vi "test-30frame-QR-static.vi"() -> ()   [LabVIEW 2015]
uses:
  <vilib>/Utility/error.llb/whitespace.ctl
  <vilib>/MakerHub/LINX/Public/Peripherals/Digital/Digital Write 1 Chan.vi
  <vilib>/MakerHub/LINX/Public/Peripherals/Analog/Analog Read N Chans.vi
  <vilib>/MakerHub/LINX/Public/Peripherals/Digital/Digital Write N Chans.vi
  <vilib>/MakerHub/LINX/Private/Local IO/LinxAnalogRead.vi
  <vilib>/MakerHub/LINX/Public/Utilities/Check Channel.vi
  <vilib>/MakerHub/LINX/Private/Local IO/LinxDigitalWrite.vi
  <vilib>/Instr/_visa.llb/VISA Configure Serial Port (Instr).vi
  <vilib>/MakerHub/LINX/Public/Utilities/Open Serial.vi
  <vilib>/MakerHub/LINX/Private/Utilties/Generate Error.vi
  <vilib>/ptbypt/NI_PtbyPt.lvlib
  <vilib>/MakerHub/LINX/LMH-LINX.lvlib
panel:
  out "gat hang 2":bool
  in  "measurement":dbl
  in  "calculate":dbl
  out "Appear":bool
  out "gat hang":bool
  in  "?":T1(tab)=enum."CONTROL & SUPERVISORY"
  in  "?":i32(listbox)
  out "Form QR ?":bool
  out "Data#":bool
  out "Found?":bool
  out "False Package":dbl
  out "SS3":bool=TRUE
  out "SS2":bool=TRUE
  out "SS1":bool=TRUE
  out "Processing Chart":cluster{dbl, dbl, dbl, dbl, "mean":dbl}(graph)={0.0, 0.0, 0.0, -16.408877733961745, "mean"=-16.408877733961745}
  out "WEIGHT PASS":bool
  out "Calculate\nValue":dbl
  out "DATA":string
  out "QR PASS":bool
  out "Well Package":i32
  out "Measurement\nValue":dbl format="%#.3f"
  in  "zero":bool
  in  "No. Accurate (g)":dbl=10.0 format="%#_13g"
  in  "Fillter":bool
  in  "STOP":bool
  in  "Start measurement":bool caption="Ðo tuyÌ choòn"
  out "CTHT1":bool=TRUE
  out "CTHT2":bool=TRUE
  in  "button CTHT 2":bool
  in  "button CTHT 1":bool
  in  "button SS 3":bool
  in  "button SS 2":bool
  in  "button SS 1":bool
  out "Trigger1":bool
  out "Trigger 2":bool
  out "?":T2(plugin-control)
  out "S/N":string
  out "C/N":string
  out "Run Loop":i32=777
  in  "Sensor Channels":u8[](array[numeric])=[4, 5, 6, 0, 1]
  in  "Path save data report":path=path "C:/Data"
  in  "COM Port Controller":refnum<visa-resource-name>="COM18"
  out "Quantity":i32=35
  out "Mass (kg):":dbl=2.0
  out "Tong K/lg (kg)":dbl=70.0
  in  "VISA resource name":refnum<visa-resource-name>="COM12"
  out "Array":i32[](array[numeric])
  out "Numeric 2":i32=233
  out "Raw data":dbl
  out "Fine Data":dbl=-16.408877733961745
  in  "zero":dbl=16.408877733961745
  in  "he so calib":dbl=8.552828494462736 format="%#_12g"
  in  "Serial Settings":T3={"baud rate"=19200, "data bits"=8, "parity"=enum."None", "stop bits"=10, "flow control"=0} {"flow control" items=["None"=0, "XON/XOFF"=1, "RTS/CTS"=2, "DTR/DSR"=4]; "stop bits" items=["1.0"=10, "1.5"=15, "2.0"=20]; "data bits" min=5 max=8 step=1; "baud rate" items=["75"=75, "110"=110, "134"=134, "150"=150, "300"=300, "600"=600, "1200"=1200, "1800"=1800, "2400"=2400, "4800"=4800, "7200"=7200, "9600"=9600, "14400"=14400, "19200"=19200, "28800"=28800, "38400"=38400, "56000"=56000, "57600"=57600, "115200"=115200, "128000"=128000, "230400"=230400]}
  in  "Low factor":cluster{"1":dbl, "2":dbl, "3":dbl}={"1"=177000.0, "2"=222000.0, "3"=-207250.0}
  in  "High Factor":cluster{"1":dbl, "2":dbl, "3":dbl}={"1"=1073000.0, "2"=1137000.0, "3"=703000.0} {"3" format="%#_15f"}
  in  "Termination Character":u8=10 format="%.0x"
  in  "End Read on\n Termination Character?":bool=TRUE
  in  "index":i32
  in  "sample length":i32=100
  in  "Numeric":i32=500
  in  "Pulse pin 2":u8=7
  in  "DIR pin 2":u8=6
  out "notifier out":refnum<notifier>
  in  "V-ref-trigger":dbl=0.2 format="%#_13g"
  out "Sensors Chart":T4(graph)={"Voltages[0]"=2.9833984375, "Voltages[1]"=1.728515625, "Voltages[2]"=0.9033203125, "Voltages[3]"=4.228515625, "Voltages[4]"=4.27734375, "Voltages[5]"=0.0, "Voltages[6]"=0.0, "Voltages[7]"=0.0, "Voltages[8]"=0.0}
  in  "Enable pin 2":u8=5
  in  "Frequency (Hz) 2":u32=6400
  in  "Frequency (Hz)":u32=6400
  in  "Pulse pin":u8=4
  in  "DIR pin":u8=3
  in  "enable pin":u8=2
  # "HÊò THÔìNG KIÊÒM TRA CHÂìT LÝÕòNG ÐOìNG GOìI THUÌNG HAÌNG\n THEO MAÞ QR & ÌKHÔìI LÝÕòNG"
  # "Table Result"
  # "TEST"
  # "Sensors"
  # "Control"
  # "Weight Transmit"
  # "Motor1"
  # "Motor2"
  # "Image Processing"
  # "Report"
  # "Distance Sensors and Limit Switch"
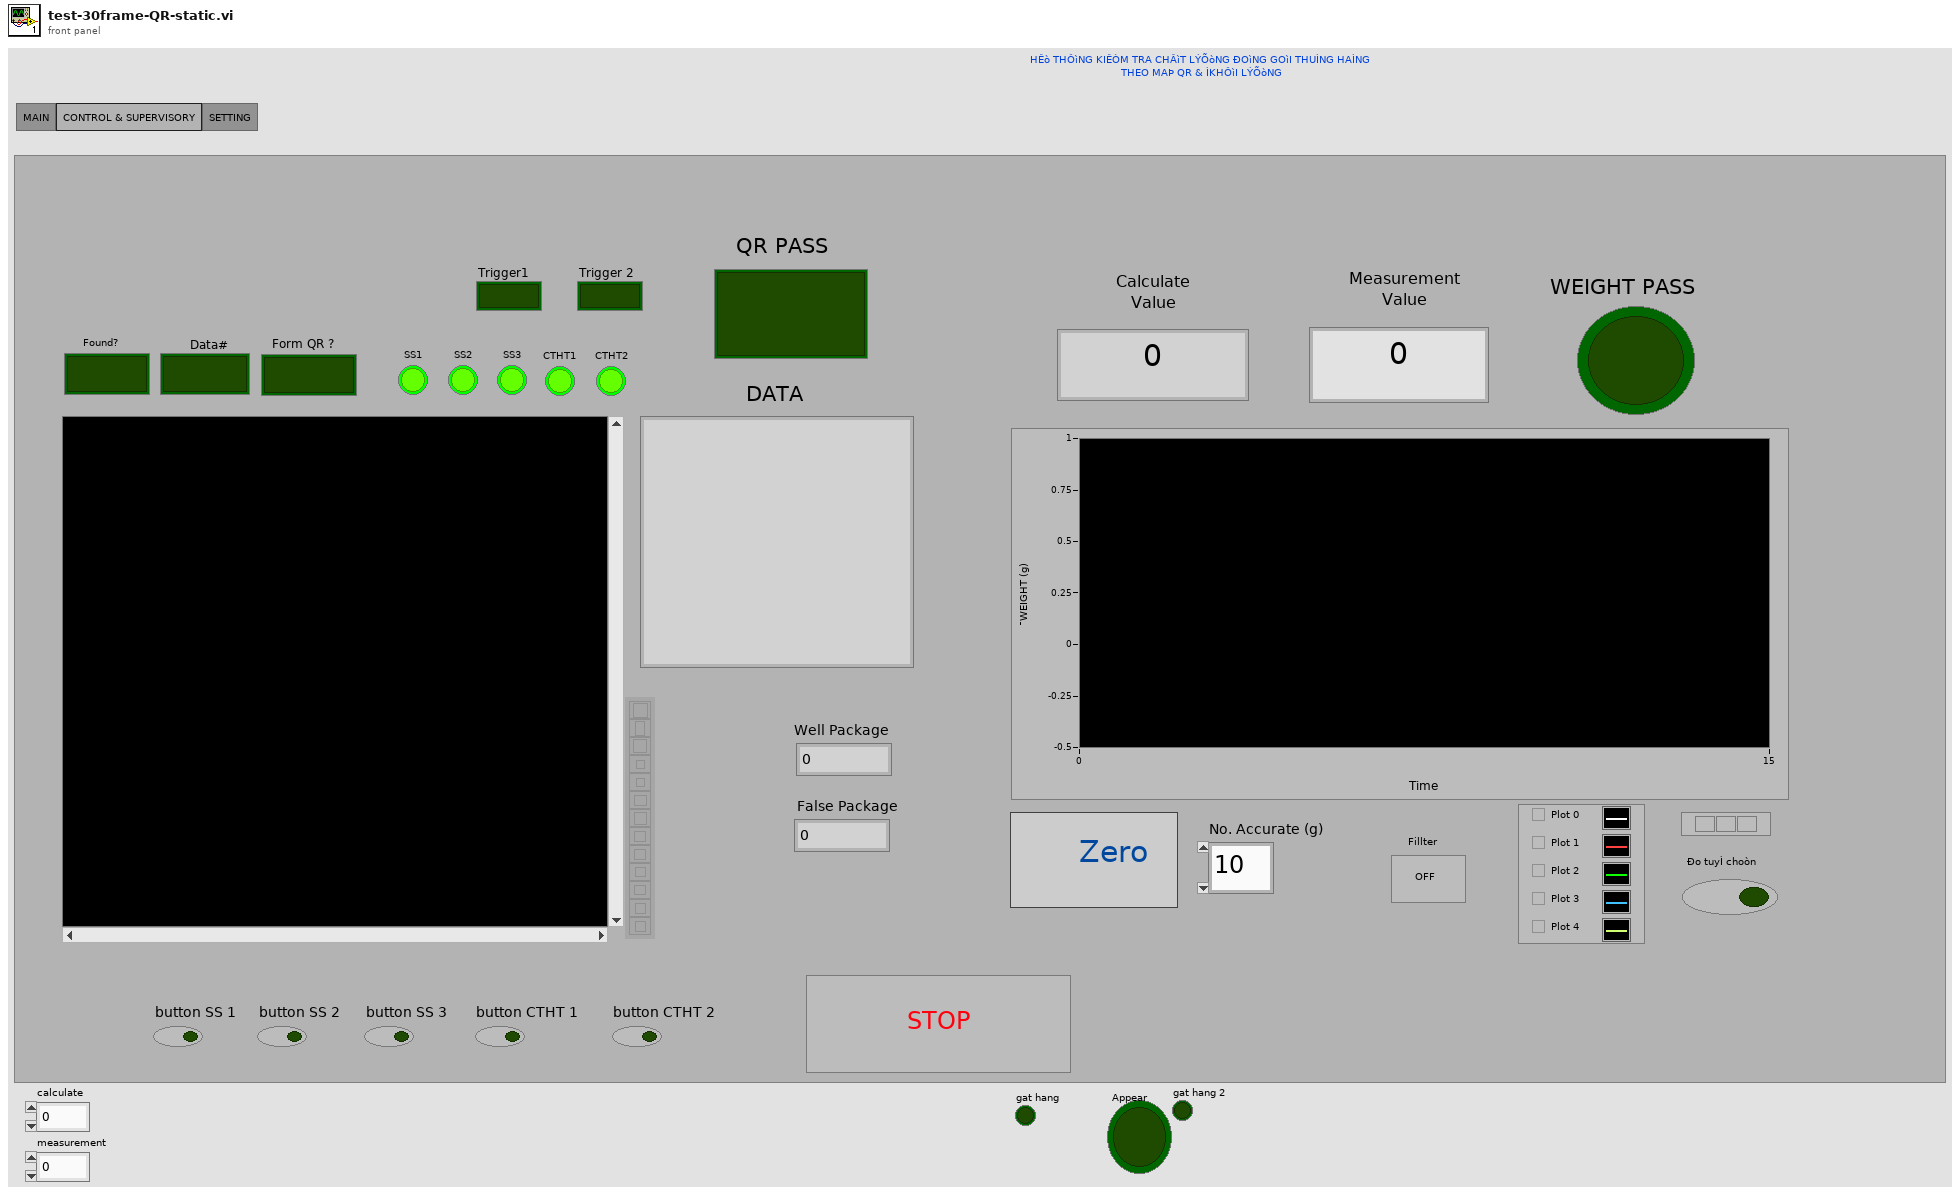
[diagram p1: front panel]
types:
  T1 = enum32{"MAIN", "CONTROL & SUPERVISORY", "SETTING"}
  T2 = typedef "IMAQ Image.ctl" = refnum<image>
  T3 = cluster{"baud rate":u32, "data bits":u16, "parity":enum16{"None", "Odd", "Even", "Mark", "Space"}, "stop bits":u16, "flow control":u16}
  T4 = cluster{"Voltages[0]":dbl, "Voltages[1]":dbl, "Voltages[2]":dbl, "Voltages[3]":dbl, "Voltages[4]":dbl, "Voltages[5]":dbl, "Voltages[6]":dbl, "Voltages[7]":dbl, "Voltages[8]":dbl}
  T5 = typedef "LMH-LINX.lvlib/LINX Ref.ctl" = cluster{"IO":T6, "Interface":T7, "LINX Device Config":T8}
  T6 = typedef "LMH-LINX.lvlib/Platform.ctl" = enum16{"Remote", "Local"}
  T7 = typedef "LMH-LINX.lvlib/Interface.ctl" = enum16{"Serial", "TCP"}
  T8 = typedef "LMH-LINX.lvlib/Device.lvlib/LINX Device Config.ctl" = cluster{"Interface":T7, "COM Port":refnum<visa-resource-name>, "TCP Configuration":T9, "Device Family":u8, "Device ID":u8, "Device Name":string, "TCP Ref":refnum<k5>, "Channels":T10}
  T9 = typedef "LMH-LINX.lvlib/Device.lvlib/TCP Config.ctl" = cluster{"IP Address":string, "Port":u16}
  T10 = typedef "LMH-LINX.lvlib/Channels.ctl" = cluster{"DI":u8[], "DO":u8[], "AI":u8[], "AO":u8[], "PWM":u8[], "QE":u8[], "UART":u8[], "I2C 2":u8[], "SPI":u8[], "CAN":u8[], "Servo":u8[], "AI Ref (V)":dbl, "AI Resolution (Bits)":u8, "AO Ref (V)":dbl, "AO Resolution (Bits)":u8}
  T11 = typedef "whitespace.ctl" = u16
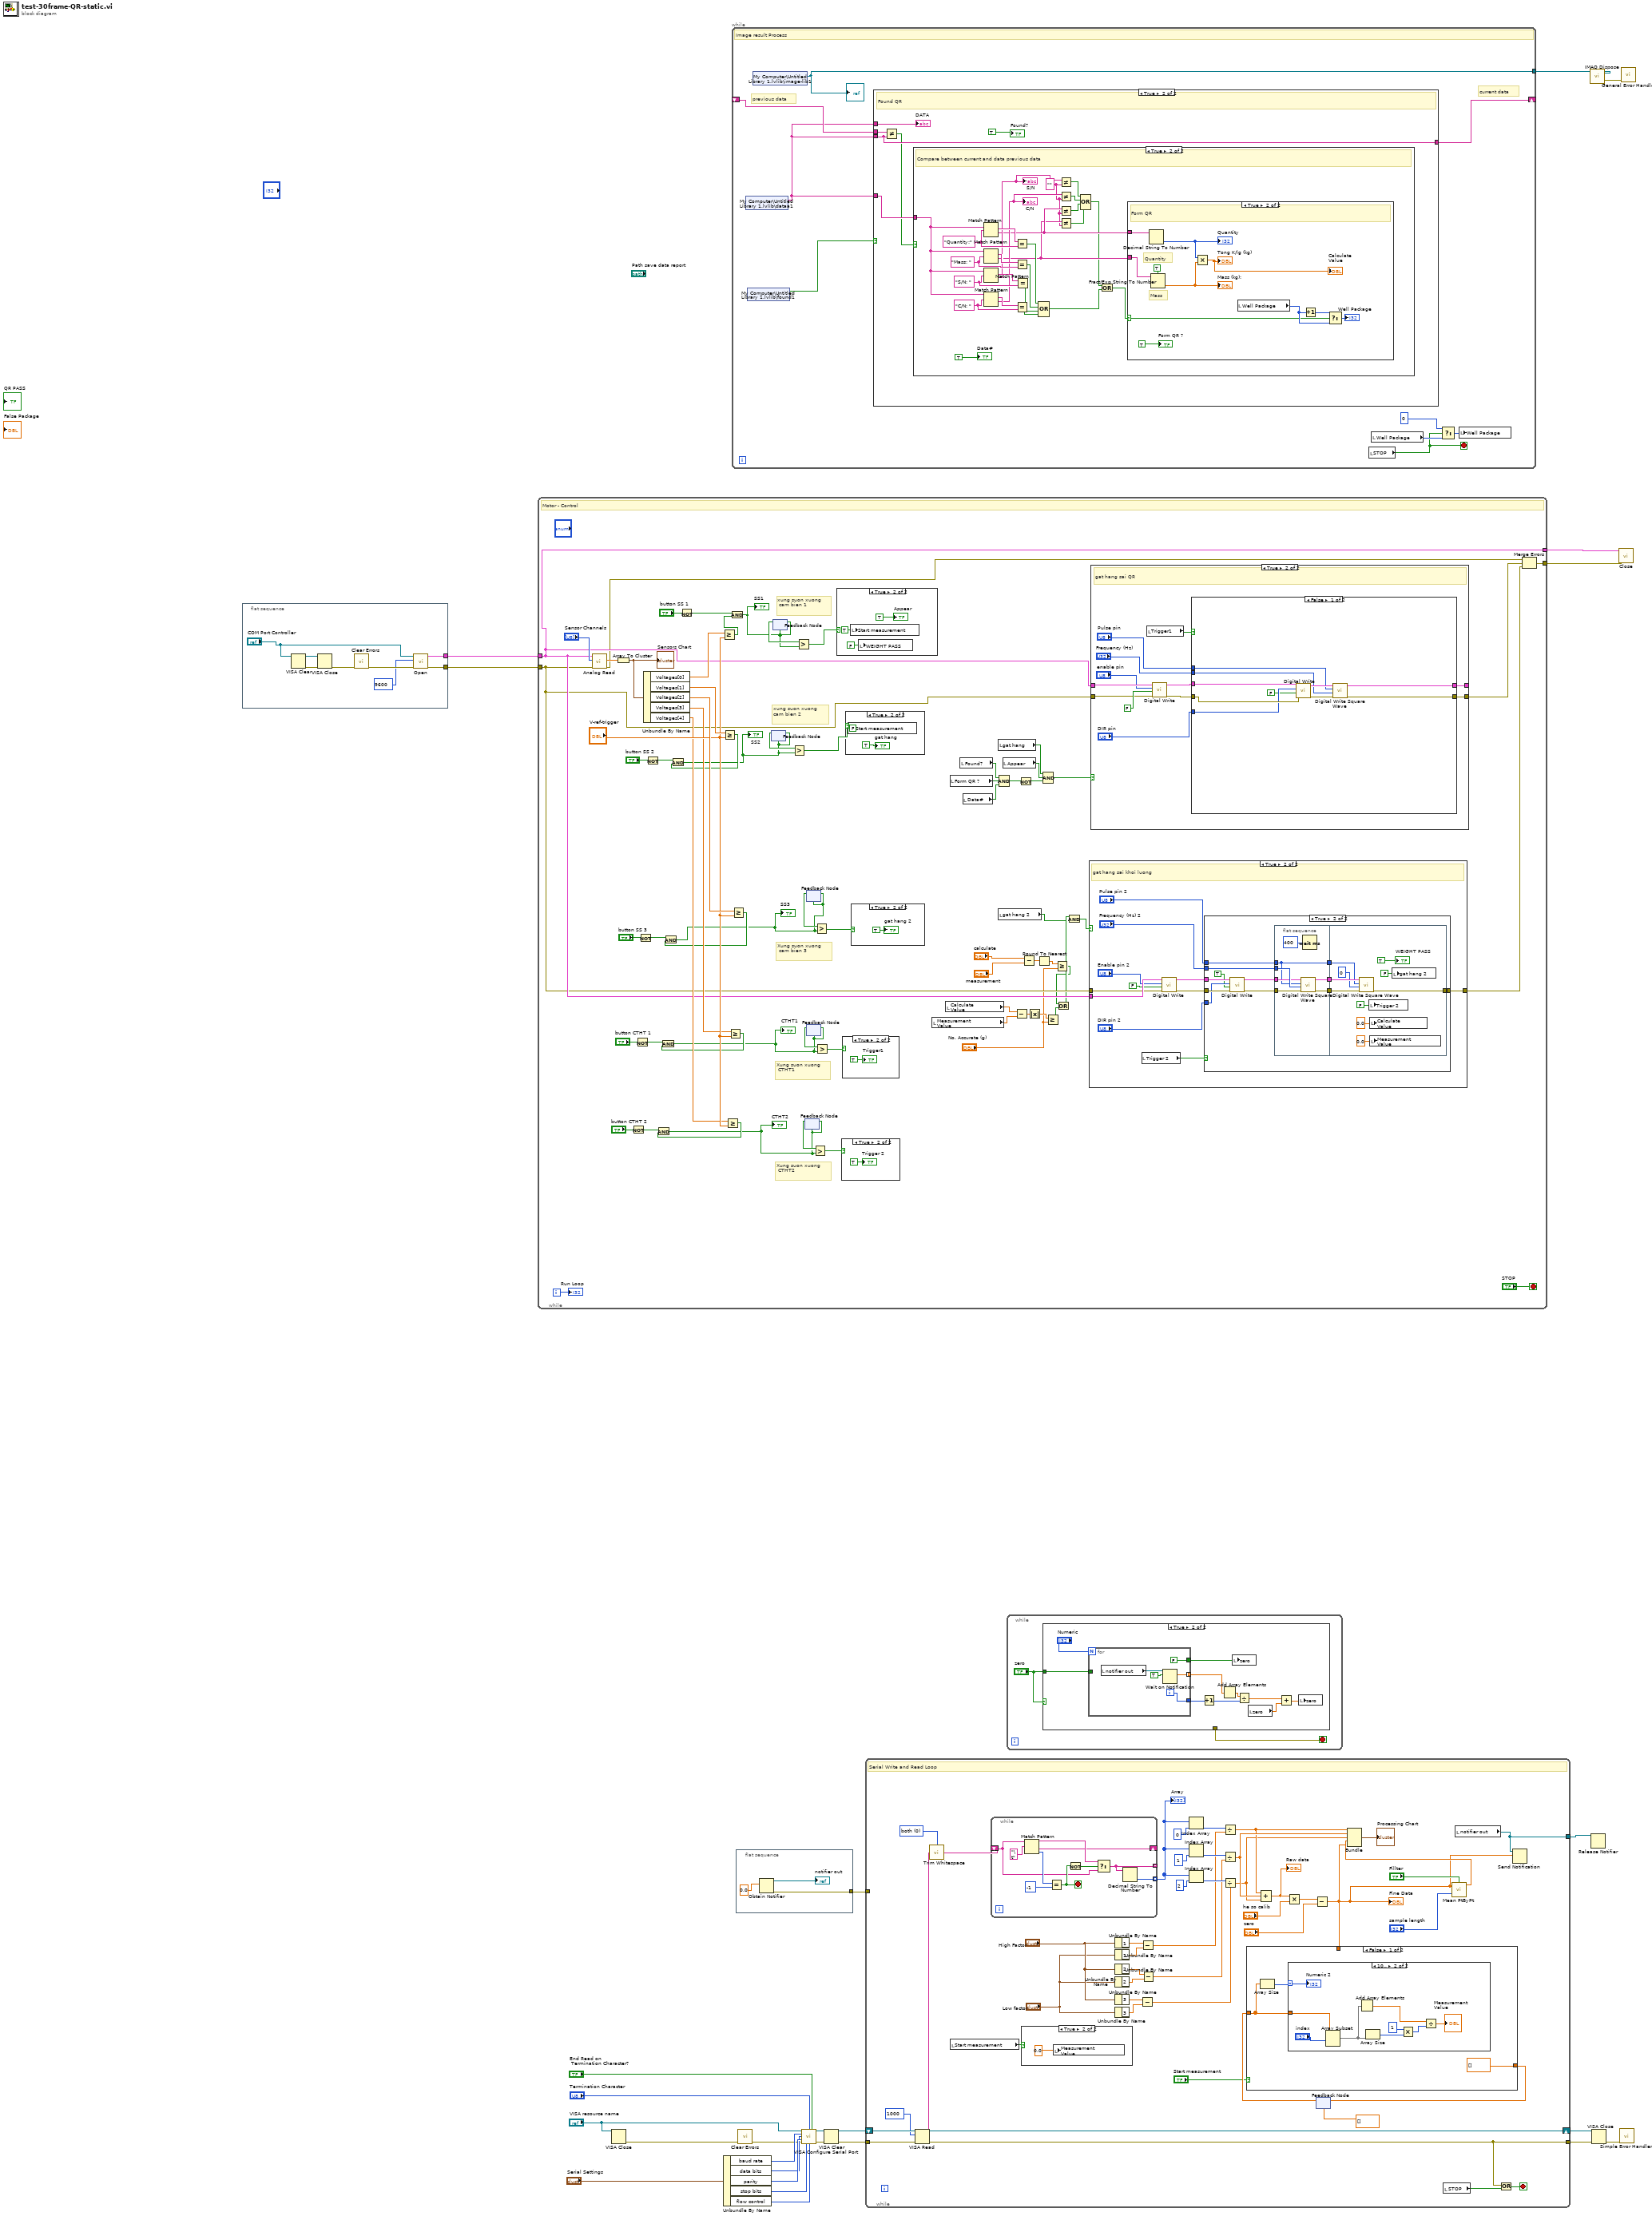
[diagram p0: block diagram]
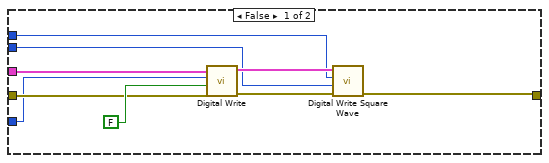
[diagram p7: hidden frame]
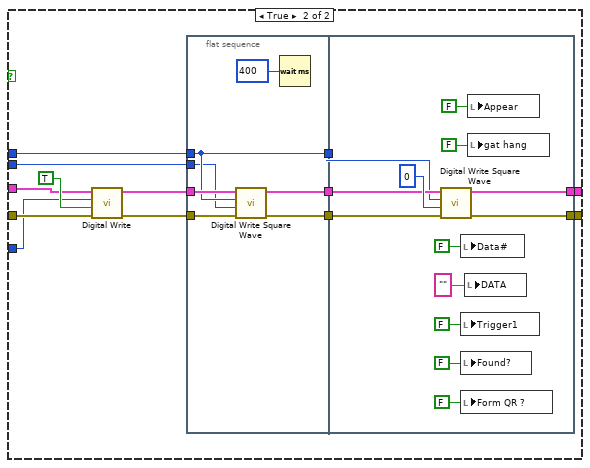
[diagram p11: hidden frame]
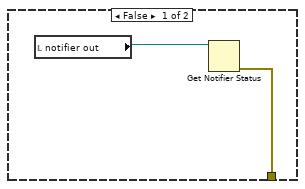
[diagram p14: hidden frame]
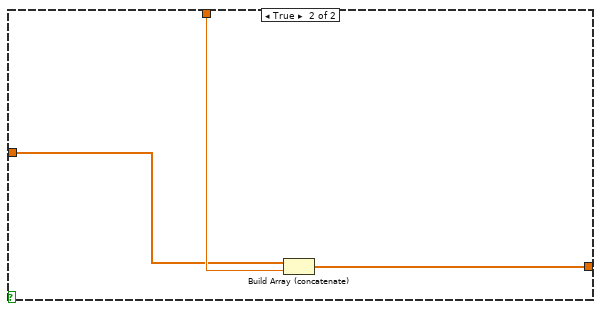
[diagram p17: hidden frame]
diagram:
  n1 = flat-sequence {
    tunnel: [w32] -> w2
    tunnel: [w31] -> w1
    frame #0 {
      n2 = VISA Clear(VISA resource name="COM Port Controller") -> (VISA resource name out=w29:refnum<visa-resource-name>, error out=w27:errorcluster)  [unwired: 1 in]
      n3 = VISA Close(VISA resource name=w29, error in (no error)=w27) -> (error out=w34:errorcluster)
      n4 = call <vilib>:"Clear Errors.vi"("error in (no error)"=w34) -> ("error out"=w33:errorcluster)  [unwired: 5 in, 1 out]
      n5 = call-poly <vilib>:"Open.vi"("Error In"=w33, "Baud Rate Override"=u32 9600, "Serial Port"="COM Port Controller") -> ("Error Out"=w31:errorcluster, "LINX Resource"=w32:T5)  [unwired: 6 in, 1 out]
    }
  }
  n6 = while {
    tunnel: w2 -> [w61]
    tunnel: w1 -> [w60]
    tunnel: [w56] -> w4
    tunnel: [w61] -> w3
    i -> [w101]
    stop <- "STOP" stop-if-true
    # "Xung suon xuong\n CTHT2"
    # "Xung suon xuong\n CTHT1"
    # "xung suon xuong\n cam bien 1"
    # "Xung suon xuong\n cam bien 3"
    # "xung suon xuong \ncam bien 2"
    # "Motor - Control"
    n7 = call-poly <vilib>:"Analog Read.vi"("Error In"=w60, "AI Channel(s)"="Sensor Channels", "LINX Resource"=w61) -> ("Error Out"=w55:errorcluster, "Voltages"=w103:dbl[])  [unwired: 5 in, 2 out]
    n8 = Array To Cluster(array=w103) -> (cluster=w92:T4)
    "Sensors Chart" <- w92
    n9 = Not(x="button CTHT 2") -> (.not. x?=w74:bool)
    n10 = Not(x="button CTHT 1") -> (.not. x?=w76:bool)
    n11 = Not(x="button SS 3") -> (.not. x?=w80:bool)
    n12 = Unbundle By Name(w92) -> ("Voltages[0]"=w99:dbl, "Voltages[1]"=w98:dbl, "Voltages[2]"=w97:dbl, "Voltages[3]"=w88:dbl, "Voltages[4]"=w87:dbl)
    n13 = Not(x="button SS 2") -> (.not. x?=w82:bool)
    n14 = Not(x="button SS 1") -> (.not. x?=w84:bool)
    n15 = Greater Or Equal?(x=w99, y="V-ref-trigger") -> (x >= y?=w86:bool)
    n16 = Greater Or Equal?(x=w98, y="V-ref-trigger") -> (x >= y?=w79:bool)
    n17 = And(x=w82, y=w79) -> (x .and. y?=w69:bool)
    "SS2" <- w69
    n18 = Greater Or Equal?(x=w87, y="V-ref-trigger") -> (x >= y?=w71:bool)
    n19 = And(x=w74, y=w71) -> (x .and. y?=w70:bool)
    "CTHT2" <- w70
    n20 = Greater Or Equal?(x=w88, y="V-ref-trigger") -> (x >= y?=w73:bool)
    n21 = And(x=w76, y=w73) -> (x .and. y?=w72:bool)
    "CTHT1" <- w72
    n22 = And(x=w84, y=w86) -> (x .and. y?=w46:bool)
    "SS1" <- w46
    n23 = Greater Or Equal?(x=w97, y="V-ref-trigger") -> (x >= y?=w78:bool)
    n24 = And(x=w80, y=w78) -> (x .and. y?=w68:bool)
    "SS3" <- w68
    n25 = feedback #1(w69) -> (w102:bool)
    n26 = feedback-in #1(w69) -> ()
    n27 = feedback #2(w46) -> (w95:bool)
    n28 = feedback-in #2(w46) -> ()
    n29 = Greater?(x=w102, y=w69) -> (0:w93:bool)
    n30 = Greater?(x=w95, y=w46) -> (0:w94:bool)
    n31 = feedback #3(w70) -> (w90:bool)
    n32 = feedback-in #3(w70) -> ()
    n33 = feedback #4(w68) -> (w96:bool)
    n34 = feedback-in #4(w68) -> ()
    n35 = feedback #5(w72) -> (w91:bool)
    n36 = feedback-in #5(w72) -> ()
    n37 = Greater?(x=w90, y=w70) -> (0:w52:bool)
    n38 = Greater?(x=w96, y=w68) -> (0:w36:bool)
    n39 = Greater?(x=w91, y=w72) -> (0:w59:bool)
    n40 = case shown="True" w94 {
      frame False {
      }
      frame True {
        n41 = local write "Start measurement"(TRUE ("bat dau do")) -> ()
        n42 = local write "WEIGHT PASS"(FALSE ("WEIGHT PASS")) -> ()
        "Appear" <- TRUE
      }
    }
    n43 = case shown="True" w52 {
      frame False {
      }
      frame True {
        "Trigger 2" <- TRUE ("Trigger 2")
      }
    }
    n44 = case shown="True" w59 {
      frame False {
      }
      frame True {
        "Trigger1" <- TRUE ("Trigger1")
      }
    }
    n45 = case shown="True" w93 {
      frame False {
      }
      frame True {
        n46 = local write "Start measurement"(FALSE ("bat dau do")) -> ()
        "gat hang" <- TRUE
      }
    }
    n47 = case shown="True" w36 {
      frame False {
      }
      frame True {
        "gat hang 2" <- TRUE ("gat hang 2")
      }
    }
    n48 = local read "Measurement\nValue"() -> (w49:dbl)
    n49 = local read "Calculate\nValue"() -> (w48:dbl)
    n50 = local read "Form QR ?"() -> (w65:bool)
    n51 = local read "Found?"() -> (w54:bool)
    n52 = local read "Data#"() -> (w66:bool)
    n53 = local read "gat hang"() -> (w63:bool)
    n54 = local read "gat hang 2"() -> (w35:bool)
    n55 = Compound Arithmetic op=AND(w54, w65, w66) -> (w64:bool)
    n56 = local read "Appear"() -> (w53:bool)
    n57 = Subtract(x=w48, y=w49) -> (x-y=w50:dbl)
    n58 = Not(x=w64) -> (.not. x?=w62:bool)
    n59 = Subtract(x="calculate", y="measurement") -> (x-y=w43:dbl)
    n60 = Absolute Value(x=w50) -> (abs(x)=w51:dbl)
    n61 = Round To Nearest(number=w43) -> (nearest integer value=w40:dbl)
    n62 = Compound Arithmetic op=AND(w63, w53, w62) -> (w58:bool)
    n63 = Greater Or Equal?(x=w51, y="No. Accurate (g)") -> (x >= y?=w45:bool)
    n64 = Greater Or Equal?(x=w40, y="No. Accurate (g)") -> (x >= y?=w38:bool)
    n65 = Or(x=w38, y=w45) -> (x .or. y?=w44:bool)
    n66 = And(x=w44, y=w35) -> (x .and. y?=w37:bool)
    n67 = case shown="True" w37 {
      tunnel: w61 -> [_ w113]
      tunnel: w60 -> [w105 w112]
      tunnel: [w105 w107] -> w47
      frame False {
      }
      frame True {
        # "gat hang sai khoi luong"
        n68 = local read "Trigger 2"() -> (w106:bool)
        n69 = call-poly <vilib>:"Digital Write.vi"("Error In"=w112, "Output Value"=FALSE, "DO Channel"="Enable pin 2", "LINX Resource"=w113) -> ("Error Out"=w108:errorcluster, "LINX Resource"=w109:T5)  [unwired: 6 in]
        n70 = case shown="True" w106 {
          tunnel: "Pulse pin 2" -> [w120 w137]
          tunnel: "DIR pin 2" -> [w118 w133]
          tunnel: "Frequency (Hz) 2" -> [w119 w136]
          tunnel: w109 -> [w122 w135]
          tunnel: w108 -> [w121 w134]
          tunnel: [w117 w127] -> w107
          frame False {
            n71 = call-poly <vilib>:"Digital Write.vi"("Error In"=w121, "Output Value"=FALSE, "DO Channel"=w118, "LINX Resource"=w122) -> ("Error Out"=w124:errorcluster, "LINX Resource"=w123:T5)  [unwired: 6 in]
            n72 = call <vilib>:"Digital Write Square Wave.vi"("Error In"=w124, "Frequency (Hz)"=w119, "Channel"=w120, "LINX Resource"=w123) -> ("Error Out"=w117:errorcluster)  [unwired: 6 in, 1 out]
          }
          frame True {
            n73 = call-poly <vilib>:"Digital Write.vi"("Error In"=w134, "Output Value"=TRUE, "DO Channel"=w133, "LINX Resource"=w135) -> ("Error Out"=w131:errorcluster, "LINX Resource"=w132:T5)  [unwired: 6 in]
            n74 = flat-sequence {
              tunnel: w137 -> [w138]
              tunnel: w136 -> [w143]
              tunnel: w132 -> [w142]
              tunnel: w131 -> [w141]
              tunnel: [w140] -> w130
              tunnel: [w139] -> w129
              tunnel: [w138] -> w128
              tunnel: w130 -> [w151]
              tunnel: w129 -> [w150]
              tunnel: w128 -> [w148]
              tunnel: [w147] -> w127
              frame #0 {
                n75 = call <vilib>:"Digital Write Square Wave.vi"("Error In"=w141, "Frequency (Hz)"=w143, "Channel"=w138, "LINX Resource"=w142) -> ("Error Out"=w139:errorcluster, "LINX Resource"=w140:T5)  [unwired: 6 in]
                n76 = Wait (ms)(milliseconds to wait=u32 400) -> ()  [unwired: 1 out]
              }
              frame #1 {
                n77 = call <vilib>:"Digital Write Square Wave.vi"("Error In"=w150, "Frequency (Hz)"=u32 0, "Channel"=w148, "LINX Resource"=w151) -> ("Error Out"=w147:errorcluster)  [unwired: 6 in, 1 out]
                n78 = local write "Trigger 2"(FALSE ("Trigger 2")) -> ()
                n79 = local write "Calculate\nValue"(0.0 ("Calculated\nValue")) -> ()
                n80 = local write "Measurement\nValue"(0.0 ("Measurement\nValue")) -> ()
                n81 = local write "gat hang 2"(FALSE ("gat hang 2")) -> ()
                "WEIGHT PASS" <- TRUE ("WEIGHT PASS")
              }
            }
          }
        }
      }
    }
    n82 = case shown="True" w58 {
      tunnel: w61 -> [w158 w167]
      tunnel: w60 -> [w157 w166]
      tunnel: [w158 w165] -> _
      tunnel: [w157 w164] -> w57
      frame False {
      }
      frame True {
        # "gat hang sai QR"
        n83 = local read "Trigger1"() -> (w163:bool)
        n84 = call-poly <vilib>:"Digital Write.vi"("Error In"=w166, "Output Value"=FALSE, "DO Channel"="enable pin", "LINX Resource"=w167) -> ("Error Out"=w168:errorcluster, "LINX Resource"=w169:T5)  [unwired: 6 in]
        n85 = case shown="False" w163 {
          tunnel: w169 -> [w180 w190]
          tunnel: w168 -> [w179 w189]
          tunnel: "DIR pin" -> [w178 w188]
          tunnel: [w177 w187] -> w165
          tunnel: [w176 w186] -> w164
          tunnel: "Pulse pin" -> [w172 w183]
          tunnel: "Frequency (Hz)" -> [w171 w181]
          frame False {
            n86 = call-poly <vilib>:"Digital Write.vi"("Error In"=w179, "Output Value"=FALSE, "DO Channel"=w178, "LINX Resource"=w180) -> ("Error Out"=w174:errorcluster, "LINX Resource"=w173:T5)  [unwired: 6 in]
            n87 = call <vilib>:"Digital Write Square Wave.vi"("Error In"=w174, "Frequency (Hz)"=w171, "Channel"=w172, "LINX Resource"=w173) -> ("Error Out"=w176:errorcluster, "LINX Resource"=w177:T5)  [unwired: 6 in]
          }
          frame True {
            n88 = call-poly <vilib>:"Digital Write.vi"("Error In"=w189, "Output Value"=TRUE, "DO Channel"=w188, "LINX Resource"=w190) -> ("Error Out"=w192:errorcluster, "LINX Resource"=w191:T5)  [unwired: 6 in]
            n89 = flat-sequence {
              tunnel: w192 -> [w200]
              tunnel: w191 -> [w199]
              tunnel: [w198] -> w185
              tunnel: [w197] -> w184
              tunnel: w183 -> [w195]
              tunnel: [w195] -> w182
              tunnel: w181 -> [w194]
              tunnel: [w209] -> w186
              tunnel: [w210] -> w187
              tunnel: w185 -> [w212]
              tunnel: w184 -> [w211]
              tunnel: w182 -> [w201]
              frame #0 {
                n90 = call <vilib>:"Digital Write Square Wave.vi"("Error In"=w200, "Frequency (Hz)"=w194, "Channel"=w195, "LINX Resource"=w199) -> ("Error Out"=w197:errorcluster, "LINX Resource"=w198:T5)  [unwired: 6 in]
                n91 = Wait (ms)(milliseconds to wait=u32 400) -> ()  [unwired: 1 out]
              }
              frame #1 {
                n92 = call <vilib>:"Digital Write Square Wave.vi"("Error In"=w211, "Frequency (Hz)"=u32 0, "Channel"=w201, "LINX Resource"=w212) -> ("Error Out"=w209:errorcluster, "LINX Resource"=w210:T5)  [unwired: 6 in]
                n93 = local write "Data#"(FALSE ("Found?")) -> ()
                n94 = local write "Trigger1"(FALSE ("Trigger1")) -> ()
                n95 = local write "Found?"(FALSE ("Form code ?")) -> ()
                n96 = local write "Form QR ?"(FALSE ("data current # data previous ?")) -> ()
                n97 = local write "DATA"("" ("data-global")) -> ()
                n98 = local write "Appear"(FALSE ("appear")) -> ()
                n99 = local write "gat hang"(FALSE ("gat hang")) -> ()
              }
            }
          }
        }
      }
    }
    n100 = Merge Errors(w55, w57, w47) -> (w56:errorcluster)
    "Run Loop" <- w101
  }
  n101 = VISA Close(VISA resource name="VISA resource name") -> (error out=w13:errorcluster)  [unwired: 1 in]
  n102 = Unbundle By Name("Serial Settings") -> ("baud rate"=w23:u32, "data bits"=w24:u16, "parity"=w25:enum16{"None", "Odd", "Even", "Mark", "Space"}, "stop bits"=w26:u16, "flow control"=w17:u16)
  n103 = while {
    shift-right: [w223] -> _
    shift-left: _ -> [w222]
    tunnel: [w219] -> w5
    stop <- w224 stop-if-true
    # "previous data"
    # "current data"
    # "Image result Process"
    n104 = shared-variable "My Computer\\Untitled Library 1.lvlib\\dataa1"() -> (w220:string)  [unwired: 1 in, 1 out]
    n105 = shared-variable "My Computer\\Untitled Library 1.lvlib\\found1"() -> (w221:bool)  [unwired: 1 in, 1 out]
    n106 = shared-variable "My Computer\\Untitled Library 1.lvlib\\image-lib1"() -> (w219:refnum<image>)  [unwired: 1 in, 1 out]
    "?" <- w219
    n107 = case shown="True" w221 {
      tunnel: w220 -> [_ w232]
      tunnel: [w228 w233] -> w223
      tunnel: w222 -> [w228 w234]
      tunnel: w220 -> [_ w233]
      tunnel: w220 -> [_ w229]
      frame False {
        # "Found QR"
      }
      frame True {
        # "Found QR"
        n108 = Not Equal?(x=w234, y=w233) -> (x != y?=w231:bool)
        n109 = case shown="True" w231 {
          tunnel: w232 -> [_ w248]
          frame False {
          }
          frame True {
            w242 = "" ("y")
            w260 = "C/N: " ("regular expression")
            w257 = "S/N: " ("regular expression")
            w255 = "Mass: " ("regular expression")
            w253 = "Quantity:" ("regular expression")
            # "Compare between current and data previous data"
            n110 = Match Pattern(string=w248, regular expression=w253) -> (match substring=w254:string, after substring=w244:string)  [unwired: 1 in, 2 out]
            n111 = Match Pattern(string=w248, regular expression=w255) -> (match substring=w256:string, after substring=w243:string)  [unwired: 1 in, 2 out]
            n112 = Match Pattern(string=w248, regular expression=w257) -> (match substring=w258:string, after substring=w246:string)  [unwired: 1 in, 2 out]
            "S/N" <- w246
            n113 = Match Pattern(string=w248, regular expression=w260) -> (match substring=w259:string, after substring=w245:string)  [unwired: 1 in, 2 out]
            "C/N" <- w245
            n114 = Equal?(x=w254, y=w253) -> (x = y?=w252:bool)
            n115 = Equal?(x=w256, y=w255) -> (x = y?=w251:bool)
            n116 = Equal?(x=w259, y=w260) -> (x = y?=w249:bool)
            n117 = Equal?(x=w258, y=w257) -> (x = y?=w250:bool)
            n118 = Compound Arithmetic op=OR(w252, w251, w250, w249) -> (w237:bool)
            n119 = Not Equal?(x=w246, y=w242) -> (x != y?=w241:bool)
            n120 = Not Equal?(x=w245, y=w242) -> (x != y?=w240:bool)
            n121 = Not Equal?(x=w244, y=w242) -> (x != y?=w239:bool)
            n122 = Not Equal?(x=w243, y=w242) -> (x != y?=w238:bool)
            n123 = Compound Arithmetic op=OR(w241, w240, w239, w238) -> (w236:bool)
            n124 = Compound Arithmetic op=OR(w236, w237) -> (w235:bool)
            n125 = case shown="True" w235 {
              selector: w235 -> [_ w263]
              tunnel: w244 -> [_ w265]
              tunnel: w243 -> [_ w264]
              frame False {
              }
              frame True {
                # "Mass"
                # "Quantity"
                # "Form QR"
                n126 = Decimal String To Number(string=w265) -> (number=w267:i32)  [unwired: 2 in, 1 out]
                "Quantity" <- w267
                n127 = Fract/Exp String To Number(use system decimal point (T)=TRUE, string=w264) -> (number=w266:dbl)  [unwired: 2 in, 1 out]
                "Mass (kg):" <- w266
                n128 = Multiply(x=w267, y=w266) -> (x*y=→"Tong K/lg (kg)" →"Calculate\nValue":dbl)
                n129 = local read "Well Package"() -> (w270:i32)
                n130 = Increment(x=w270) -> (x+1=w269:i32)
                n131 = Select(t=w269, s=w263, f=w270) -> (s? t:f=→"Well Package":i32)
                "Form QR ?" <- TRUE ("Form code ?")
              }
            }
            "Data#" <- TRUE ("data current # data previous ?")
          }
        }
        "Found?" <- TRUE ("Found?")
        "DATA" <- w229
      }
    }
    n132 = local read "STOP"() -> (w224:bool)
    n133 = local read "Well Package"() -> (w225:i32)
    n134 = Select(t=0, s=w224, f=w225) -> (s? t:f=w227:i32)
    n135 = local write "Well Package"(w227) -> ()
  }
  n136 = flat-sequence {
    tunnel: [w272] -> w8
    frame #0 {
      n137 = Obtain Notifier(notification data type=0.0 ("Y Scale.Range:Maximum")) -> (notifier out=→"notifier out":refnum<notifier>, error out=w272:errorcluster)  [unwired: 3 in, 1 out]
    }
  }
  n138 = call <vilib>:"Clear Errors.vi"("error in (no error)"=w13) -> ("error out"=w12:errorcluster)  [unwired: 5 in, 1 out]
  n139 = call-poly "VISA Configure Serial Port"("VISA resource name"="VISA resource name", "termination char\n(0xA = '\\n' = LF)"="Termination Character", "Enable Termination\nChar (T)"="End Read on\n Termination Character?", "baud rate (9600)"=w23, "data bits (8)"=w24, "parity (0:none)"=w25, "error in (no error)"=w12, "stop bits (10: 1 bit)"=w26, "flow control (0:none)"=w17) -> ("VISA resource name out"=w16:refnum<visa-resource-name>, "error out"=w10:errorcluster)  [unwired: 1 in, 4 out]
  n140 = VISA Clear(VISA resource name=w16, error in (no error)=w10) -> (VISA resource name out=w11:refnum<visa-resource-name>, error out=w9:errorcluster)
  n141 = while {
    shift-right: [w320] -> w18
    shift-left: w11 -> [w319]
    tunnel: w9 -> [w318]
    tunnel: [w317] -> w19
    tunnel: w8 -> [_]
    tunnel: [w279] -> w7
    stop <- w295 stop-if-true
    w315 = T11 0 items=["both", "start of string", "end of string"] ("location (both)")
    # "Serial Write and Read Loop"
    n142 = VISA Read(VISA resource name=w319, byte count=u32 1000 ("Read Count"), error in (no error)=w318) -> (VISA resource name out=w320:refnum<visa-resource-name>, read buffer=w299:string, error out=w317:errorcluster)  [unwired: 1 out]
    n143 = call <vilib>:"Trim Whitespace.vi"("string"=w299, "location (both)"=w315) -> ("trimmed string"=w314:string)
    n144 = local read "Start measurement"() -> (w282:bool)
    n145 = while {
      shift-right: [w341] -> _
      shift-left: w314 -> [w338]
      tunnel: [w340] -> _ mode=indexing
      tunnel: [w337] -> w300 mode=indexing
      stop <- w344 stop-if-true
      n146 = Match Pattern(string=w338, regular expression="\t") -> (before substring=w342:string, after substring=w341:string, offset past match=w346:i32)  [unwired: 1 in, 1 out]
      n147 = Equal?(x=w346, y=-1) -> (x = y?=w344:bool)
      n148 = Not(x=w344) -> (.not. x?=w343:bool)
      n149 = Select(t=w342, s=w343, f=w338) -> (s? t:f=w340:string)
      n150 = Decimal String To Number(string=w340) -> (number=w337:i32)  [unwired: 2 in, 1 out]
    }
    "Array" <- w300
    n151 = case shown="True" w282 {
      frame False {
      }
      frame True {
        n152 = local write "Measurement\nValue"(0.0 ("x/y")) -> ()
      }
    }
    n153 = Unbundle By Name "Unbundle By Name"("High Factor") -> ("1"=w294:dbl)
    n154 = Unbundle By Name("Low factor") -> ("1"=w293:dbl)
    n155 = Unbundle By Name("High Factor") -> ("2"=w291:dbl)
    n156 = Unbundle By Name("Low factor") -> ("2"=w292:dbl)
    n157 = Unbundle By Name("High Factor") -> ("3"=w290:dbl)
    n158 = Unbundle By Name("Low factor") -> ("3"=w289:dbl)
    n159 = Subtract(x=w290, y=w289) -> (x-y=w285:dbl)
    n160 = Subtract(x=w294, y=w293) -> (x-y=w287:dbl)
    n161 = Subtract(x=w291, y=w292) -> (x-y=w286:dbl)
    n162 = Index Array "Index Array"(array=w300, index=0) -> (element=w311:i32)
    n163 = Index Array(array=w300, index=1) -> (element=w310:i32)
    n164 = Index Array(array=w300, index=2) -> (element=w307:i32)
    n165 = Divide(x=w311, y=w287) -> (x/y=w306:dbl)
    n166 = Divide(x=w310, y=w286) -> (x/y=w309:dbl)
    n167 = Divide(x=w307, y=w285) -> (x/y=w305:dbl)
    n168 = Compound Arithmetic op=ADD(w306, w309, w305) -> (w304:dbl)
    "Raw data" <- w304
    n169 = Multiply(x=w304, y="he so calib") -> (x*y=w302:dbl)
    n170 = Subtract(x=w302, y="zero") -> (x-y=w275:dbl)
    "Fine Data" <- w275
    n171 = feedback #6(dbl[] []) -> (w296:dbl[])
    n172 = case shown="False" "Start measurement" {
      tunnel: w275 -> [_ w336]
      tunnel: [dbl[] [] w335] -> w297
      tunnel: w296 -> [w322 w334]
      frame False {
        n173 = Array Size(array=w322) -> (size(s)=w323:i32)
        n174 = case shown="10.." w323 {
          selector: w323 -> [_ w332]
          tunnel: w322 -> [_ w330]
          frame 0, Default {
          }
          frame 10.. {
            n175 = Array Subset(array=w330, index="index") -> (w328:dbl[])  [unwired: 1 in]
            n176 = Add Array Elements(numeric array=w328) -> (sum=w333:dbl)
            n177 = Array Size(array=w328) -> (size(s)=w327:i32)
            n178 = Multiply(x=1, y=w327) -> (x*y=w326:i32)
            n179 = Divide(x=w333, y=w326) -> (x/y=→"Measurement\nValue":dbl)
            "Numeric 2" <- w332
          }
        }
      }
      frame True {
        n180 = Build Array (concatenate) "Build Array"(w334, w336) -> (w335:dbl[])
      }
    }
    n181 = feedback-in #6(w297) -> ()
    n182 = local read "STOP"() -> (w278:bool)
    n183 = call <vilib>:"Mean PtByPt.vi"("x"=w275, "sample length"="sample length", "initialize"="Fillter") -> ("mean"=w276:dbl)  [unwired: 1 in, 1 out]
    n184 = Bundle(w306, w309, w305, "mean"=w276, w275) -> (→"Processing Chart":cluster{dbl, dbl, dbl, "mean":dbl, dbl})  [unwired: 1 in]
    n185 = local read "notifier out"() -> (w279:refnum<notifier>)
    n186 = Or(x=w317, y=w278) -> (x .or. y?=w295:bool)
    n187 = Send Notification(notification=w275, notifier=w279) -> ()  [unwired: 1 in, 2 out]
  }
  n188 = while {
    stop <- w347 stop-if-true
    n189 = case shown="True" "zero" {
      tunnel: "zero" -> [_ w360]
      tunnel: [w349 _] -> w347
      frame False {
        n190 = local read "notifier out"() -> (w350:refnum<notifier>)
        n191 = Get Notifier Status(notifier=w350) -> (error out=w349:errorcluster)  [unwired: 1 in, 4 out]
      }
      frame True {
        n192 = for {
          N: "Numeric" -> [_]
          tunnel: w360 -> [_]
          tunnel: [FALSE ("zero")] -> w359
          tunnel: [w362] -> w355 mode=indexing
          tunnel: [w361] -> w353
          i -> [w361]
          n193 = local read "notifier out"() -> (w365:refnum<notifier>)
          n194 = Wait on Notification(notifier=w365, ignore previous (F)=TRUE) -> (notification=w362:dbl)  [unwired: 2 in, 3 out]
        }
        n195 = Increment(x=w353) -> (x+1=w352:i32)
        n196 = Add Array Elements(numeric array=w355) -> (sum=w354:dbl)
        n197 = local write "zero"(w359) -> ()
        n198 = Divide(x=w354, y=w352) -> (x/y=w351:dbl)
        n199 = local read "zero"() -> (w357:dbl)
        n200 = Add(x=w351, y=w357) -> (x+y=w356:dbl)
        n201 = local write "zero"(w356) -> ()
      }
    }
  }
  n202 = call "IMAQ Dispose"("Image"=w5) -> ("error out"=w6:errorcluster)  [unwired: 5 in]
  n203 = Release Notifier(notifier=w7) -> ()  [unwired: 2 in, 3 out]
  n204 = VISA Close(VISA resource name=w18, error in (no error)=w19) -> (error out=w20:errorcluster)
  n205 = call <vilib>:"Close.vi"("Error In"=w4, "LINX Resource"=w3) -> ()  [unwired: 9 in, 1 out]
  n206 = call <vilib>:"Simple Error Handler.vi"("error in (no error)"=w20) -> ()  [unwired: 1 in, 8 out]
  n207 = call <vilib>:"General Error Handler.vi"("error in (no error)"=w6) -> ()  [unwired: 10 in, 5 out]
